vi "AddToVisited.vi"(8 "error in (no error)":errorcluster, 9 "Path":path, 11 "CVisitedSet in":refnum<class "CVisitedSet.lvclass">) -> (0 "error out":errorcluster, 3 "CVisitedSet out":refnum<class "CVisitedSet.lvclass">)   [LabVIEW 2020, in "DependencyInspection.lvlib" / "CVisitedSet.lvclass"]
uses:
  CVisitedSet.lvclass
  CVisitedSet.lvclass/CVisitedSet.ctl
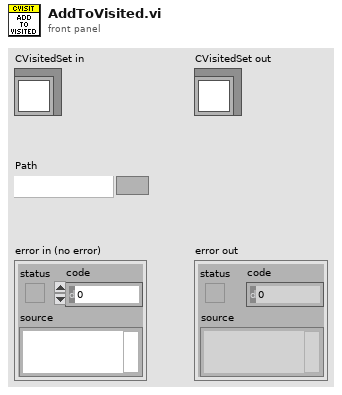
[diagram p1: front panel]
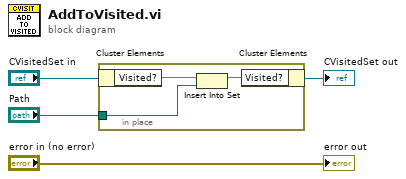
[diagram p0: block diagram]
diagram:
  n1 = in-place {
    in-place-border: "Path" -> [w5]
    n2 = in-place-cluster #1("CVisitedSet in") -> ("Visited?"=w7:set{path})
    n3 = Insert Into Set(10:w5, 11:w7) -> (3:w6:set{path})  [unwired: 1 out]
    n4 = in-place-cluster #1("Visited?"=w6) -> (→"CVisitedSet out":refnum<class "CVisitedSet.lvclass">)
  }
  "error out" <- "error in (no error)"
